vi "Reader List Item to Reader Name.vi"() -> (0 "Reader Name":string)   [LabVIEW 2017, in "Scan Driver.lvclass"]
uses:
  Scan Driver.lvclass
  Reader List.ctl
panel:
  in  "Reader List Item":T1
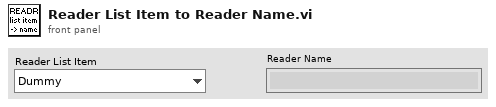
[diagram p1: front panel]
types:
  T1 = typedef "Scan Driver.lvclass/Reader List.ctl" = enum16{"Dummy", "Cryostat Temperature", "DAQmx Analog", "Lockin SR830", "Multimeter", "Photon Counter", "Power Meter", "Temperature Control"}
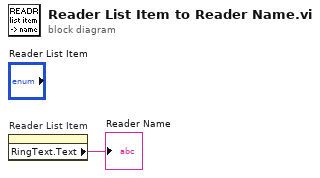
[diagram p0: block diagram]
diagram:
  n1 = property on="Reader List Item" class="Enum (strict)"() -> ("RingText.Text"=→"Reader Name":string)  [unwired: 2 in, 2 out]
